vi "Mexa_One_string-to-array.vi"(4 "Array in":string[](array[string])) -> (1 "Array out":dbl[](array[numeric]))   [LabVIEW 2014]
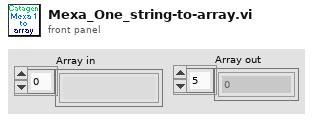
[diagram p1: front panel]
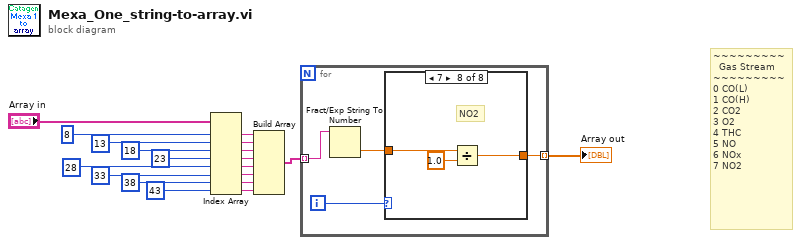
[diagram p0: block diagram]
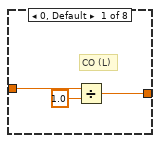
[diagram p2: hidden frame]
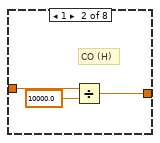
[diagram p3: hidden frame]
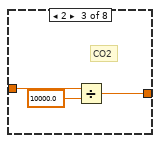
[diagram p4: hidden frame]
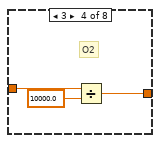
[diagram p5: hidden frame]
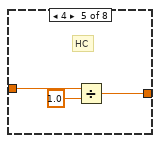
[diagram p6: hidden frame]
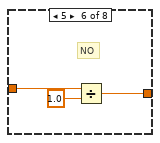
[diagram p7: hidden frame]
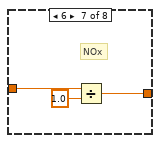
[diagram p8: hidden frame]
diagram:
  # "~~~~~~~~~  \n  Gas Stream\n~~~~~~~~~\n0 CO(L)\n1 CO(H)\n2 CO2\n3 O2\n4 THC\n5 NO\n6 NOx\n7 NO2"
  n1 = Index Array(array="Array in", index #1=8 ("index"), index #2=13 ("index"), index #3=18 ("index"), index #4=23 ("index"), index #5=28 ("index"), index #6=33 ("index"), index #7=38 ("index"), index #8=43 ("index")) -> (element #1=w11:string, element #2=w10:string, element #3=w9:string, element #4=w8:string, element #5=w7:string, element #6=w6:string, element #7=w5:string, element #8=w1:string)
  n2 = Build Array(w11, w10, w9, w8, w7, w6, w5, w1) -> (w4:string[])
  n3 = for {
    tunnel: w4 -> [w22] mode=indexing
    tunnel: [w20] -> w3 mode=indexing
    i -> [w23]
    n4 = Fract/Exp String To Number(string=w22) -> (number=w21:dbl)  [unwired: 3 in, 1 out]
    n5 = case shown="7" w23 {
      tunnel: w21 -> [w24 w29 w30 w33 w36 w39 w42 w45]
      tunnel: [w25 w27 w31 w34 w37 w40 w43 w46] -> w20
      frame 0, Default {
        # "CO (L)"
        n6 = Divide(x=w24, y=1.0) -> (x/y=w25:dbl)
      }
      frame 1 {
        # "CO (H)"
        n7 = Divide(x=w29, y=10000.0) -> (x/y=w27:dbl)
      }
      frame 2 {
        # "CO2"
        n8 = Divide(x=w30, y=10000.0) -> (x/y=w31:dbl)
      }
      frame 3 {
        # "O2"
        n9 = Divide(x=w33, y=10000.0) -> (x/y=w34:dbl)
      }
      frame 4 {
        # "HC"
        n10 = Divide(x=w36, y=1.0) -> (x/y=w37:dbl)
      }
      frame 5 {
        # "NO"
        n11 = Divide(x=w39, y=1.0) -> (x/y=w40:dbl)
      }
      frame 6 {
        # "NOx"
        n12 = Divide(x=w42, y=1.0) -> (x/y=w43:dbl)
      }
      frame 7 {
        # "NO2"
        n13 = Divide(x=w45, y=1.0) -> (x/y=w46:dbl)
      }
    }
  }
  "Array out" <- w3
